vi "Load Credentials.vi"() -> (0 "error out":errorcluster, 2 "Key":string, 3 "ID":string)   [LabVIEW 2024, in "Wordle Scorer.lvlib"]
uses:
  Wordle Scorer.lvlib
  <vilib>/Utility/config.llb/NI_LVConfig.lvlib
  <vilib>/Utility/config.llb/Read Key (String).vi
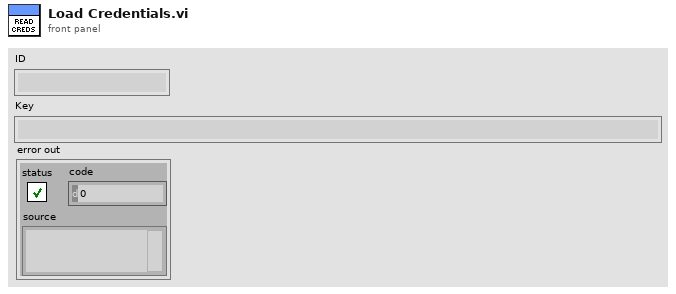
[diagram p1: front panel]
types:
  T1 = typedef "NI_LVConfig.lvlib/Config Data RefNum.ctl" = refnum<k1>
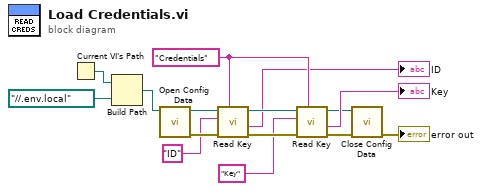
[diagram p0: block diagram]
diagram:
  w6 = "Credentials" ("section")
  n1 = Current VI's Path() -> (path=w15:path)
  n2 = Build Path(base path=w15, name or relative path=path "../../.env.local") -> (appended path=w13:path)
  n3 = call <vilib>:"Open Config Data.vi"("configuration file path"=w13) -> ("error out"=w12:errorcluster, "refnum"=w11:T1)  [unwired: 8 in, 1 out]
  n4 = call-poly <vilib>:"Read Key.vi"("section"=w6, "error in (no error)"=w12, "key"="ID", "refnum"=w11) -> ("error out"=w9:errorcluster, "value"=→"ID":string, "refnum out"=w8:T1)  [unwired: 4 in, 1 out]
  n5 = call-poly <vilib>:"Read Key.vi"("section"=w6, "error in (no error)"=w9, "key"="Key", "refnum"=w8) -> ("error out"=w2:errorcluster, "value"=→"Key":string, "refnum out"=w3:T1)  [unwired: 4 in, 1 out]
  n6 = call <vilib>:"Close Config Data.vi"("error in (no error)"=w2, "refnum"=w3) -> ("error out"=→"error out":errorcluster)  [unwired: 8 in, 1 out]
